vi "Initialize Session.vi"(5 "Password":string, 6 "Connect Timeout (4000 ms)":u32=4000, 7 "User Name":string, 8 "error in (no error)":errorcluster, 9 "Language (Automatic)":T1 items=["Automatic"=0, "Chinese Simplified"=2052, "English"=1033, "French"=1036, "German"=1031, "Japanese"=1041, "Korean"=1042], 10 "Force Property Refresh (T)":bool=TRUE, 11 "Target (localhost)":refnum<k21>="localhost") -> (0 "error out":errorcluster, 3 "Session out":refnum<k21>)   [LabVIEW 2020, in "nisyscfg.lvlib"]
doc: "Initializes any system configuration VI to gather information from a specified target. You must use this VI to obtain a handle for a specified target that can be used in other System Configuration VIs.\n\n<B>NOTE:</B> This VI communicates to the device at the specified address. If the device is no longer online, but it has previously been discovered in Measurement & Automation Explorer (MAX), this VI succeeds, allowing you to retrieve cached information about the device. To determine if a Real-Time target is online, use the System Property Node to return the System Status property."
uses:
  <vilib>/nisyscfg/nisyscfg.lvlib
  <vilib>/nisyscfg/Language.ctl
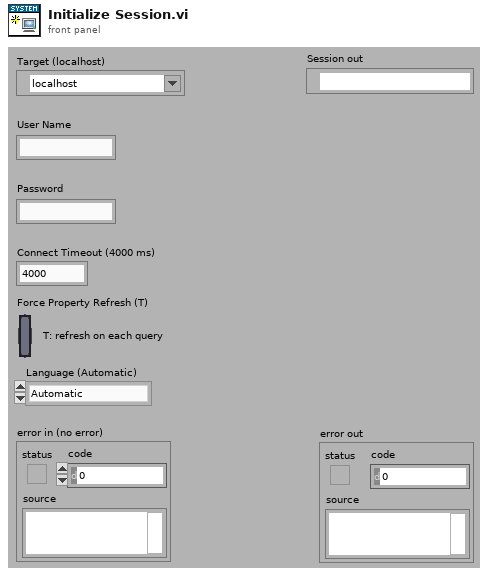
[diagram p1: front panel]
types:
  T1 = typedef "nisyscfg.lvlib/Language.ctl" = i32
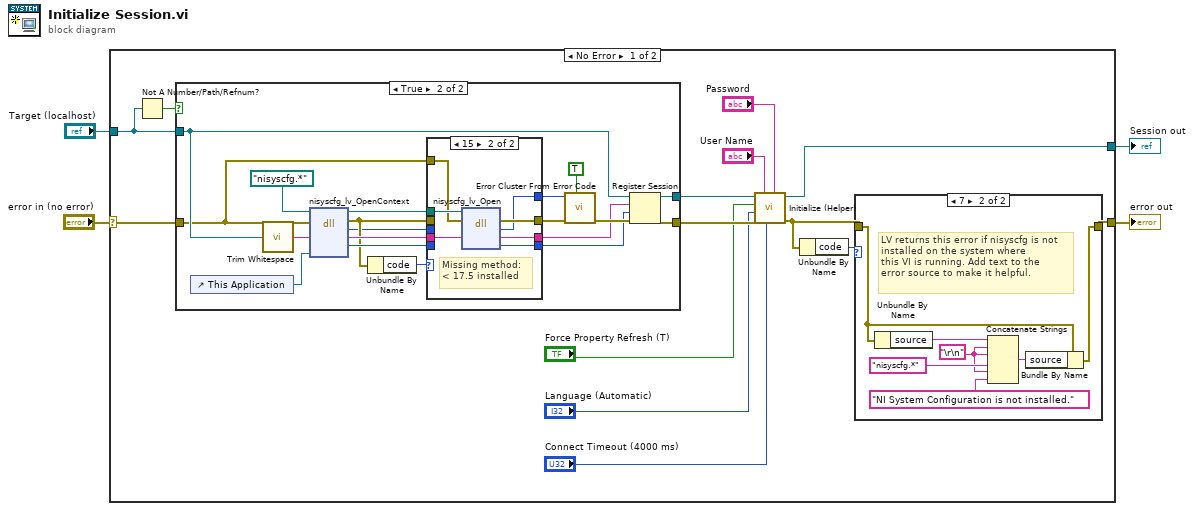
[diagram p0: block diagram]
diagram:
  n1 = case shown="No Error" "error in (no error)" {
    selector: "error in (no error)" -> [w12 w60]
    tunnel: [w6 w60] -> w4
    tunnel: [w11 w59] -> w2
    tunnel: "Target (localhost)" -> [w17 w59]
    frame No Error {
      n2 = Not A Number/Path/Refnum?(number/path/refnum=w17) -> (NaN/Path/Refnum?=w18:bool)
      n3 = case shown="True" w18 {
        tunnel: w12 -> [w27 w32]
        tunnel: [w27 w47] -> w16
        tunnel: [w28 w46] -> w13
        tunnel: w17 -> [w28 w45]
        frame False {
        }
        frame True {
          n4 = control-ref of="This Application"() -> (w41:refnum<vi>)
          n5 = call <vilib>:"Trim Whitespace.vi"("string"=w45) -> ("trimmed string"=w43:string)  [unwired: 1 in]
          n6 = dll-call lib="nisyscfg.*" fn="nisyscfg_lv_OpenContext" label="OpenContext"(path in=path "nisyscfg.*", error in=w32, "target"=w43, "appReference"=w41) -> (path out=w33:path, error out=w31:errorcluster, "status"=w29:i32, "target"=w40:string, "sessionHandle"=w39:u64)  [unwired: 1 in, 2 out]
          n7 = Unbundle By Name(w31) -> ("code"=w30:i32)
          n8 = case shown="15" w30 {
            tunnel: w31 -> [w51 _]
            tunnel: w40 -> [w50 w54]
            tunnel: w39 -> [w49 _]
            tunnel: [w51 w58] -> w38
            tunnel: [w50 w56] -> w37
            tunnel: [w49 w57] -> w36
            tunnel: [w48 w55] -> w35
            tunnel: w33 -> [_ w53]
            tunnel: w32 -> [_ w52]
            tunnel: w29 -> [w48 _]
            frame Default {
            }
            frame 15 {
              # "Missing method:\n< 17.5 installed"
              n9 = dll-call lib="nisyscfg.*" fn="nisyscfg_lv_Open" label="Open"(path in=w53, error in=w52, "target"=w54) -> (error out=w58:errorcluster, "status"=w55:i32, "target"=w56:string, "sessionHandle"=w57:u64)  [unwired: 1 in, 2 out]
            }
          }
          n10 = call <vilib>:"Error Cluster From Error Code.vi"("show call chain? (False)"=TRUE, "error in (no error)"=w38, "error code (0)"=w35) -> ("error out"=w44:errorcluster)  [unwired: 6 out]
          n11 = Register Session(8:w44, 9:w36, 10:w37, 11:w45) -> (0:w47:errorcluster, 3:w46:refnum<k21>)  [unwired: 1 in]
        }
      }
      n12 = call <vilib>:"Initialize (Helper).vi"("Password"="Password", "Connect Timeout (4000 ms)"="Connect Timeout (4000 ms)", "User Name"="User Name", "error in (no error)"=w16, "Language (Automatic)"="Language (Automatic)", "Force Property Refresh (T)"="Force Property Refresh (T)", "Session in"=w13) -> ("error out"=w7:errorcluster, "Session out"=w11:refnum<k21>)  [unwired: 3 in]
      n13 = Unbundle By Name(w7) -> ("code"=w8:i32)
      n14 = case shown="7" w8 {
        tunnel: w7 -> [w19 w26]
        tunnel: [w19 w25] -> w6
        frame Default {
        }
        frame 7 {
          w21 = "\r\n"
          # "LV returns this error if nisyscfg is not\ninstalled on the system where\nthis VI is running. Add text to the\nerror source to make it helpful."
          n15 = Unbundle By Name(w26) -> ("source"=w23:string)
          n16 = Concatenate Strings(w23, w21, w21, "nisyscfg.*", w21, "NI System Configuration is not installed.") -> (w24:string)
          n17 = Bundle By Name(cluster=w26, "source"=w24) -> (w25:errorcluster)
        }
      }
    }
    frame Error {
    }
  }
  "error out" <- w4
  "Session out" <- w2
